vi "Test.vi"() -> ()   [LabVIEW 2010]
uses:
  TrialBasedExperimentObject/TrialBasedExperiment.lvclass
  Trial Based Experiment.lvsc/Inputs.ctl
  <vilib>/Statechart/Infrastructure/RTStatechart/RunTime SCN.xnode
  Trial Based Experiment.lvsc/Outputs.ctl
  Trial Based Experiment.lvsc
  <vilib>/Statechart/Common/IntGuid.ctl
  <vilib>/Statechart/Common/DbgID.ctl
  Trial Based Experiment.lvsc/CompanionDiagram.vi/153/SC Main.vi
  <vilib>/Statechart/Common/NI_SC_LVSCCommonFiles.lvlib
panel:
  in  "Stop":bool
  in  "Pause":bool
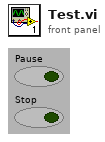
[diagram p1: front panel]
types:
  T1 = typedef "Trial Based Experiment.lvsc/Inputs.ctl" = cluster{"Timing":cluster{"Intertrial time":dbl, "Acquire fixation time":dbl, "Hold fixation time":dbl, "Delay period time":dbl, "Response time":dbl, "Reward":dbl, "Punish time":dbl}, "Stop":bool, "Control states":cluster{"Fixated":bool, "Centered":bool}, "Pause":bool, "Hammer running":bool, "Experiment":refnum<class "TrialBasedExperiment.lvclass">}
  T2 = typedef "NI_SC_LVSCCommonFiles.lvlib/IntGuid.ctl" = cluster{"Data1":u32, "Data2":u16, "Data3":u16, "Data4":u8, "Data5":u8, "Data6":u8, "Data11":u8, "Data9":u8, "Data10":u8, "Data8":u8, "Data7":u8}
  T3 = typedef "NI_SC_LVSCCommonFiles.lvlib/DbgID.ctl" = cluster{"VIRef":u32, "IntGUID":T2}
  T4 = typedef "Trial Based Experiment.lvsc/Outputs.ctl" = cluster{"Experiment":refnum<class "TrialBasedExperiment.lvclass">, "Timeout":dbl}
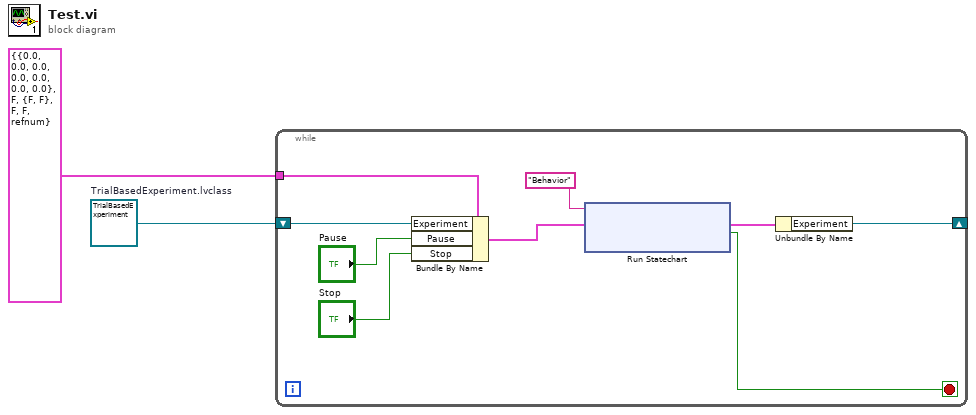
[diagram p0: block diagram]
diagram:
  w2 = refnum<class "TrialBasedExperiment.lvclass"> refnum  # TrialBasedExperiment.lvclass
  n1 = while {
    tunnel: T1 {"Timing"={"Intertrial time"=0.0, "Acquire fixation time"=0.0, "Hold fixation time"=0.0, "Delay period time"=0.0, "Response time"=0.0, "Reward"=0.0, "Punish time"=0.0}, "Stop"=FALSE, "Control states"={"Fixated"=FALSE, "Centered"=FALSE}, "Pause"=FALSE, "Hammer running"=FALSE, "Experiment"=refnum} ("Inputs") -> [w9]
    shift-right: [w6] -> _
    shift-left: w2 -> [w10]
    stop <- w3 stop-if-true
    n2 = Bundle By Name(cluster=w9, "Experiment"=w10, "Pause"="Pause", "Stop"="Stop") -> (w8:T1)
    n3 = xnode "Run Statechart"("Inputs"=w8, "Instance Name"="Behavior") -> ("Terminated?"=w3:bool, "Outputs"=w7:T4)  [unwired: 1 in]
    n4 = Unbundle By Name(w7) -> ("Experiment"=w6:refnum<class "TrialBasedExperiment.lvclass">)
  }
